vi "Get Linker Errors.vi"(8 "error in (no error)":errorcluster, 11 "EXE in":refnum<class "NI_AB_API_EXE.lvclass">) -> (0 "error out":errorcluster, 2 "Missing VIs Call Chain":variant, 3 "EXE out":refnum<class "NI_AB_API_EXE.lvclass">, 5 "Has errors?":bool)   [LabVIEW 2020, in "NI_AB_API_EXE.lvclass"]
uses:
  <vilib>/AppBuilder/AB_API/EXE/NI_AB_API_EXE.lvclass
  <vilib>/AppBuilder/AB_API/Application/NI_AB_API_Application.lvclass
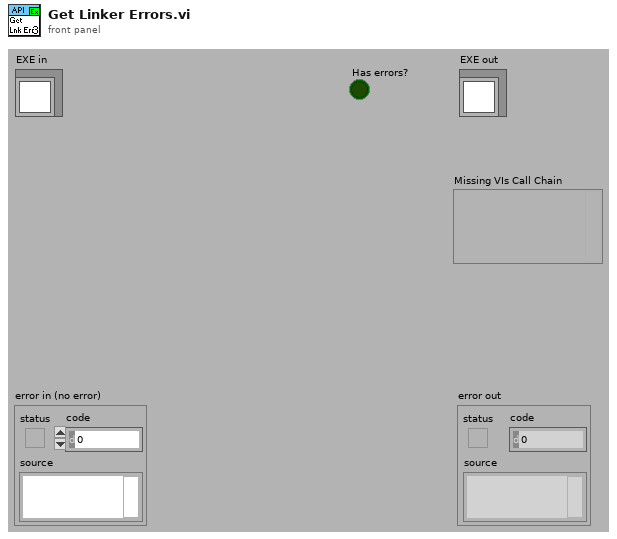
[diagram p1: front panel]
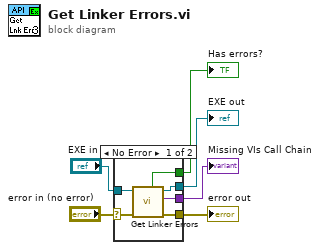
[diagram p0: block diagram]
diagram:
  n1 = case shown="No Error" "error in (no error)" {
    selector: "error in (no error)" -> [w9 w14]
    tunnel: [w10 w14] -> w5
    tunnel: [w11 w13] -> w3
    tunnel: "EXE in" -> [w12 w13]
    tunnel: [w8 _] -> w2
    tunnel: [w7 _] -> w1
    frame No Error {
      n2 = call-parent "Get Linker Errors.vi"("error in (no error)"=w9, "NI_AB_API_Build in"=w12) -> ("error out"=w10:errorcluster, "Missing VIs Call Chain"=w7:variant, "NI_AB_API_Build out"=w11:refnum<class "NI_AB_API_EXE.lvclass">, "Has errors?"=w8:bool)  [unwired: 6 in]
    }
    frame Error {
    }
  }
  "error out" <- w5
  "EXE out" <- w3
  "Has errors?" <- w2
  "Missing VIs Call Chain" <- w1
